vi "Thermometer (Demo).vi"(10 "Units (0: Celsius)":u16(ring) items=["Celsius", "Fahrenheit"]) -> (1 "Temperature Value":dbl(slide) scale=0.0..100.0)   [LabVIEW 2012]
doc: "This VI simulates measuring a temperature using the temperature sensor on the DAQ BNC-2120 terminal block.\n\nIf you have a DAQ board connected to the BNC-2120 and have configured the system in MAX, then use the Thermometer VI instead."
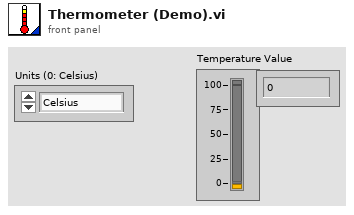
[diagram p1: front panel]
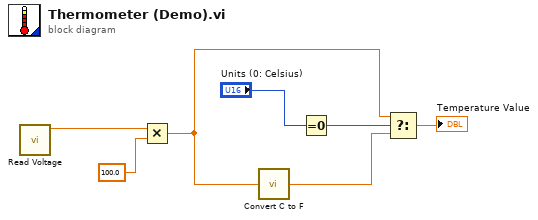
[diagram p0: block diagram]
diagram:
  n1 = call "Read Voltage.vi"() -> ("Voltage"=w4:dbl)  [unwired: 8 in, 1 out]
  n2 = Multiply(x=w4, y=100.0) -> (x*y=w5:dbl)
  n3 = call "Convert C to F.vi"("Degrees Celsius"=w5) -> ("Degrees Fahrenheit"=w7:dbl)
  n4 = Equal To 0?(x="Units (0: Celsius)") -> (x = 0?=w1:bool)
  n5 = Select(t=w5, s=w1, f=w7) -> (s? t:f=→"Temperature Value":dbl)
